vi "GetVIActivationDVR.vi"(8 "error in (no error)":errorcluster, 11 "VIActivation in":refnum<class "VIActivation.lvclass">) -> (0 "error out":errorcluster, 2 "DVR":refnum<data-value>, 3 "VIActivation out":refnum<class "VIActivation.lvclass">)   [LabVIEW 2021]
uses:
  data.ctl
  VIActivation.lvclass
  C:/Users/Dany/OneDrive/LabVIEW/Class/ClassUtilities/ClassByRef/ClassByRef.lvclass
  C:/Users/Dany/OneDrive/LabVIEW/Class/VIActivation/VIActivation.lvclass
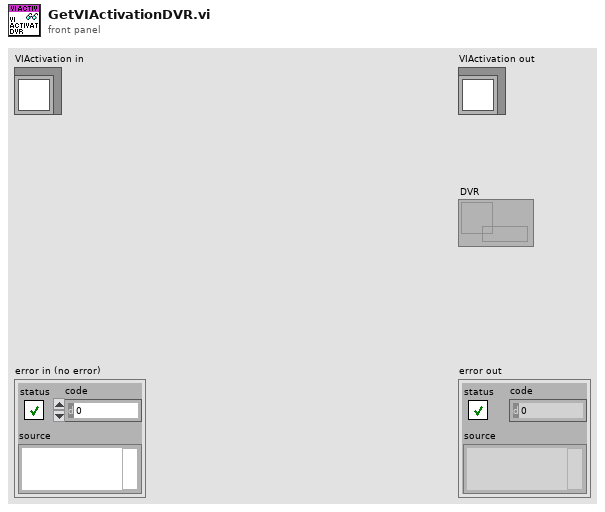
[diagram p1: front panel]
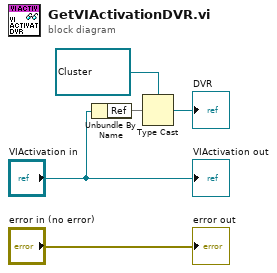
[diagram p0: block diagram]
diagram:
  n1 = Unbundle By Name("VIActivation in") -> ("Ref"=w1)
  n2 = Type Cast(type=refnum<data-value> refnum ("DVR"), x=w1) -> (*(type *) &x=→"DVR":refnum<data-value>)
  "error out" <- "error in (no error)"
  "VIActivation out" <- "VIActivation in"
